vi "sub_trigger-checkforstart.vi"(7 "check":enum16{"check", "clear"}(ring), 11 "caFwf":waveform(dbl)[](array[waveform])) -> (0 "result array":bool[](array[boolean]), 1 "stop trg":bool, 2 "start trg":bool, 3 "trigger":bool)   [LabVIEW 2013]
uses:
  <vilib>/Analysis/baseanly.llb/Mean (DBL).vi
  <vilib>/measure/mamon.llb/Trigger Detection for 1 Channel.vi
  <vilib>/measure/NI_MAPro.lvlib
  <vilib>/Analysis/NI_AALBase.lvlib
panel:
  in  "trg flag":cluster{"start":bool, "stop":bool, "high":bool}
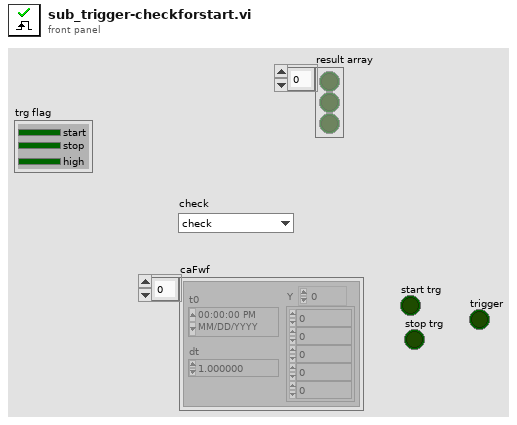
[diagram p1: front panel]
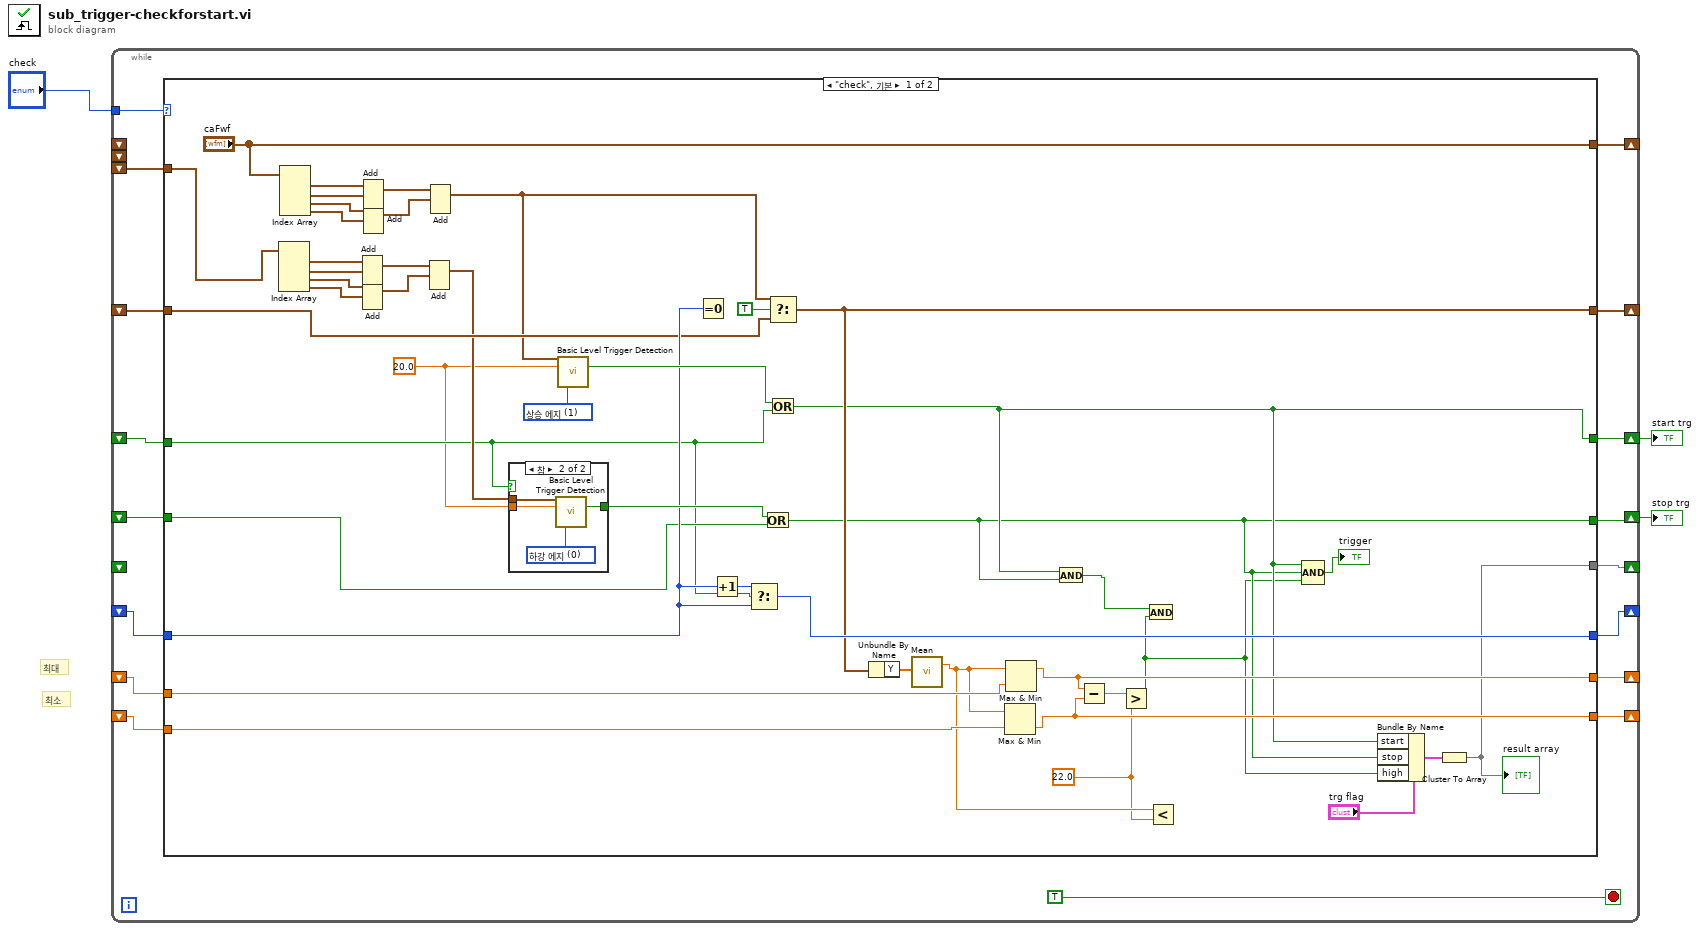
[diagram p0: block diagram]
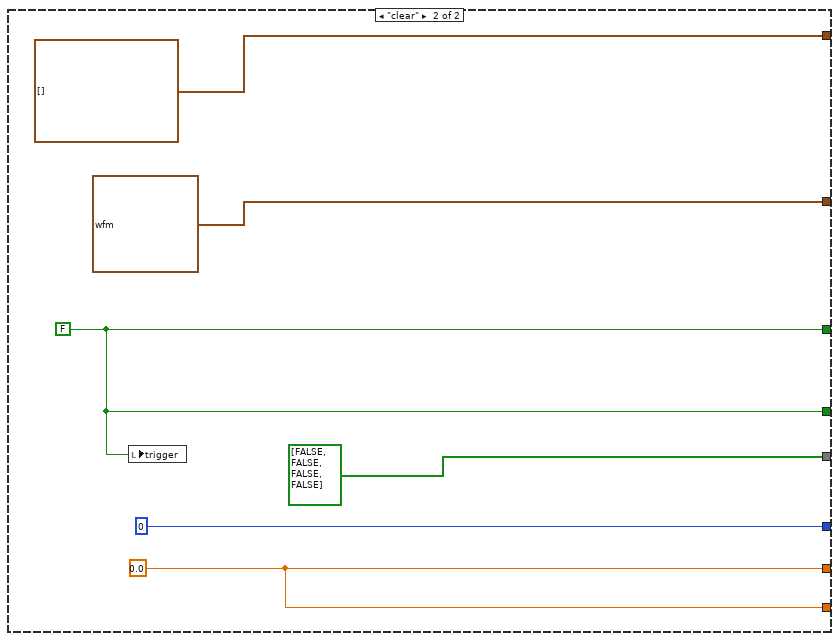
[diagram p3: hidden frame]
diagram:
  # "최소"
  # "최대"
  n1 = while {
    shift-right: [w18] -> w2
    shift-left: _ -> [w17]
    tunnel: "check" -> [w19]
    shift-right: [w16] -> _
    shift-left: _ -> [_]
    shift-left: _ -> [_]
    shift-left: _ -> [w15]
    shift-right: [w14] -> w1
    shift-left: _ -> [w13]
    shift-right: [w11] -> _
    shift-left: _ -> [w12]
    shift-right: [w10] -> _
    shift-left: _ -> [w9]
    shift-right: [w6] -> _
    shift-left: _ -> [w8]
    shift-right: [w5] -> _
    shift-left: _ -> [w7]
    shift-right: [w4] -> _
    shift-left: _ -> [_]
    stop <- TRUE stop-if-true
    n2 = case shown="\"check\", 기본" w19 {
      tunnel: [w26 w71] -> w18
      tunnel: w17 -> [w42 _]
      tunnel: ["caFwf" waveform(dbl)[] [] ("caFwf")] -> w16
      tunnel: w15 -> [w41 _]
      tunnel: [w25 w71] -> w14
      tunnel: w13 -> [w45 _]
      tunnel: w12 -> [w47 _]
      tunnel: [w48 0] -> w11
      tunnel: [w40 waveform(dbl) {"t0"=timestamp(0 s since 1904-01-01), "dt"=1.0, "Y"=[]} ("Waveform")] -> w10
      tunnel: w9 -> [w46 _]
      tunnel: w8 -> [w37 _]
      tunnel: w7 -> [w36 _]
      tunnel: [w35 w70] -> w6
      tunnel: [w34 w70] -> w5
      tunnel: [w21 bool[] [FALSE, FALSE, FALSE, FALSE]] -> w4
      frame "check", Default {
        w22 = 20.0 ("level")
        w29 = 22.0 ("y")
        w52 = u16 1 items=["하강 에지", "상승 에지"] ("trigger slope")
        n3 = Index Array(array=w41) -> (element #1=w55:waveform(dbl), element #2=w56:waveform(dbl), element #3=w57:waveform(dbl), element #4=w58:waveform(dbl))  [unwired: 4 in]
        n4 = Index Array(array="caFwf") -> (element #1=w62:waveform(dbl), element #2=w61:waveform(dbl), element #3=w60:waveform(dbl), element #4=w59:waveform(dbl))  [unwired: 4 in]
        n5 = Add(1:w56, 2:w55) -> (0:w54:waveform(dbl))  [unwired: 1 in, 1 out]
        n6 = Add(1:w58, 2:w57) -> (0:w53:waveform(dbl))  [unwired: 1 in, 1 out]
        n7 = Add(1:w61, 2:w62) -> (0:w63:waveform(dbl))  [unwired: 1 in, 1 out]
        n8 = Add(1:w59, 2:w60) -> (0:w64:waveform(dbl))  [unwired: 1 in, 1 out]
        n9 = Add(1:w53, 2:w54) -> (0:w44:waveform(dbl))  [unwired: 1 in, 1 out]
        n10 = Add(1:w64, 2:w63) -> (0:w39:waveform(dbl))  [unwired: 1 in, 1 out]
        n11 = case shown="참" w42 {
          tunnel: [_ w67] -> w50
          tunnel: w44 -> [_ w66]
          tunnel: w22 -> [_ w65]
          frame False {
          }
          frame True {
            w68 = u16 0 items=["하강 에지", "상승 에지"] ("trigger slope")
            n12 = call-poly <vilib>:"Basic Level Trigger Detection.vi"("signal in"=w66, "level"=w65, "trigger slope"=w68) -> ("trigger detected?"=w67:bool)  [unwired: 10 in, 2 out]
          }
        }
        n13 = call-poly <vilib>:"Basic Level Trigger Detection.vi"("signal in"=w39, "level"=w22, "trigger slope"=w52) -> ("trigger detected?"=w51:bool)  [unwired: 10 in, 2 out]
        n14 = Equal To 0?(x=w47) -> ()  [unwired: 1 out]
        n15 = Increment(x=w47) -> (x+1=w49:i32)
        n16 = Select(t=w49, s=w42, f=w47) -> (s? t:f=w48:i32)
        n17 = Or(x=w50, y=w45) -> (x .or. y?=w25:bool)
        n18 = Select(t=w39, s=TRUE, f=w46) -> (s? t:f=w40:waveform(dbl))
        n19 = Or(x=w51, y=w42) -> (x .or. y?=w26:bool)
        n20 = Unbundle By Name(w40) -> ("Y"=w38:dbl[])
        n21 = call-poly <vilib>:"Mean.vi"("X"=w38) -> ("mean"=w30:dbl)  [unwired: 1 out]
        n22 = Max & Min(x=w30, y=w36) -> (min(x,y)=w34:dbl)  [unwired: 1 out]
        n23 = Max & Min(x=w30, y=w37) -> (max(x,y)=w35:dbl)  [unwired: 1 out]
        n24 = And(x=w26, y=w25) -> (x .and. y?=w32:bool)
        n25 = Subtract(x=w35, y=w34) -> (x-y=w33:dbl)
        n26 = Greater?(x=w33, y=w29) -> (0:w24:bool)
        n27 = And(x=w32, y=w24) -> ()  [unwired: 1 out]
        n28 = Less?(x=w30, y=w29) -> ()  [unwired: 1 out]
        n29 = Compound Arithmetic op=AND(w26, w25, w24) -> (→"trigger":bool)
        n30 = Bundle By Name(cluster="trg flag", "start"=w26, "stop"=w25, "high"=w24) -> (w23:cluster{"start":bool, "stop":bool, "high":bool})
        n31 = Cluster To Array(cluster=w23) -> (array=w21:bool[])
        "result array" <- w21
      }
      frame "clear" {
        w70 = 0.0
        w71 = FALSE
        n32 = local write "trigger"(w71) -> ()
      }
    }
  }
  "start trg" <- w2
  "stop trg" <- w1
